vi "Servo Command.vi"(8 "Servo Period (ms)":dbl min=-100.0 max=100.0, 11 "IO Cluster IN":T1) -> (0 "Error Out":errorcluster, 3 "IO Cluster OUT":T1)   [LabVIEW 2019]
uses:
  Actuators IO Cluster.ctl
  <vilib>/Utility/error.llb/Error Cluster From Error Code.vi
  <vilib>/rvi/errors/niLvFpgaAdjustHostInterfaceError.vi
  <vilib>/rvi/interface/nirviReadWriteControl/nirviReadWriteControl.xnode
  NiFpgaLv.dll
  <vilib>/rvi/interface/Simulation/niFpgaSimulationCallBeginRW.vi
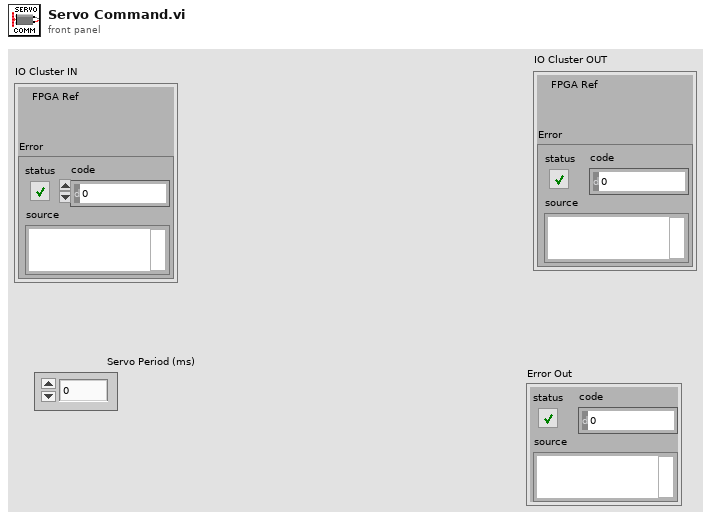
[diagram p1: front panel]
types:
  T1 = typedef "Actuators IO Cluster.ctl" = cluster{"Error":errorcluster, "FPGA Ref":refnum<k20>}
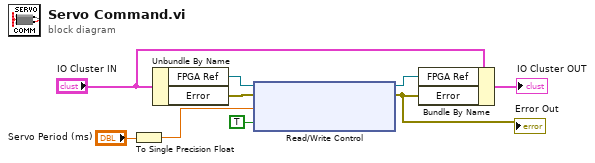
[diagram p0: block diagram]
diagram:
  n1 = To Single Precision Float(number="Servo Period (ms)") -> (single precision float=w1:sgl)
  n2 = Unbundle By Name("IO Cluster IN") -> ("FPGA Ref"=w6:refnum<k20>, "Error"=w5:errorcluster)
  n3 = xnode "Read/Write Control"("FPGA VI引用输入"=w6, "错误输入"=w5, "Servo Period (1-2ms)"=w1, "LED Servo"=TRUE) -> ("FPGA VI引用输出"=w8:refnum<k20>, "错误输出"=w7:errorcluster)
  "Error Out" <- w7
  n4 = Bundle By Name(cluster="IO Cluster IN", "FPGA Ref"=w8, "Error"=w7) -> (→"IO Cluster OUT":T1)
